vi "Color to RGB.vi"(11 "1D Pixel Array":u32[](array[numeric])) -> (1 "Blue[]":u8[](array[numeric]), 2 "Green[]":u8[](array[numeric]), 3 "Red[]":u8[](array[numeric]))   [LabVIEW 2014, in "Image Comparison.lvclass"]
uses:
  Image Comparison.lvclass
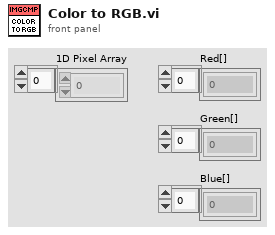
[diagram p1: front panel]
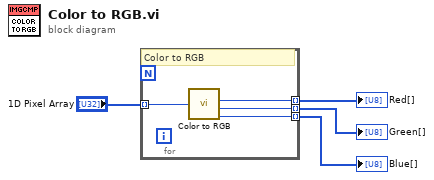
[diagram p0: block diagram]
diagram:
  n1 = for {
    tunnel: "1D Pixel Array" -> [w8] mode=indexing
    tunnel: [w7] -> w2 mode=indexing
    tunnel: [w6] -> w3 mode=indexing
    tunnel: [w5] -> w4 mode=indexing
    # "Color to RGB"
    n2 = call <vilib>:"Color to RGB.vi"("Color"=w8) -> ("R"=w7:u8, "G"=w6:u8, "B"=w5:u8)  [unwired: 1 out]
  }
  "Blue[]" <- w4
  "Green[]" <- w3
  "Red[]" <- w2
